vi "Add Dependency Dialog.vi"() -> (1 "Cancelled?":bool, 3 "Dependency Out":T3)   [LabVIEW 2015, in "Configuration Tool.lvlib"]
uses:
  XML Controls/Dependencies Properties.ctl
  XML Controls/Path Cluster.ctl
  XML Controls/Supported Targets.ctl
  Configuration Tool.lvlib
  VeriStand Custom Device XML Parser.lvlib
panel:
  in  "Cancel_Button":bool
  in  "OK_Button":bool
  in  "Path Properties":T1
  in  "Supported Target":T2
  in  "Supported Target Specified?":bool
  in  "Version":string
  in  "RealTimeSystemDestination":string
  in  "Force Download":bool
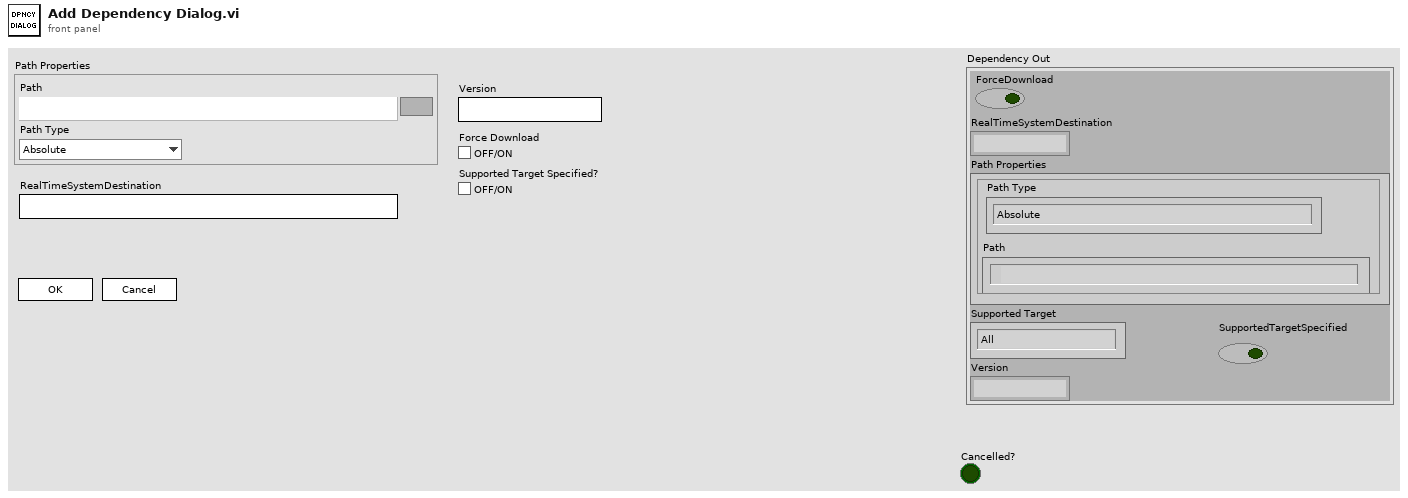
[diagram p1: front panel]
types:
  T1 = typedef "VeriStand Custom Device XML Parser.lvlib/Path Cluster.ctl" = cluster{"Path":path, "Path Type":enum16{"Absolute", "To Base", "To Common Doc Dir", "To Application Data Dir"}}
  T2 = typedef "VeriStand Custom Device XML Parser.lvlib/Supported Targets.ctl" = enum16{"All", "Pharlap", "VxWorks", "Windows", "Linux_32_ARM", "Linux_x64", "PharlapWindows", "PharlapVxWorks", "VxWorksWindows"}
  T3 = typedef "VeriStand Custom Device XML Parser.lvlib/Dependencies Properties.ctl" = cluster{"ForceDownload":bool, "RealTimeSystemDestination":string, "Path Properties":T1, "Supported Target":T2, "Version":string, "SupportedTargetSpecified":bool}
  T4 = enum32{"Invalid", "Standard", "Closed", "Hidden", "Minimized", "Maximized"}
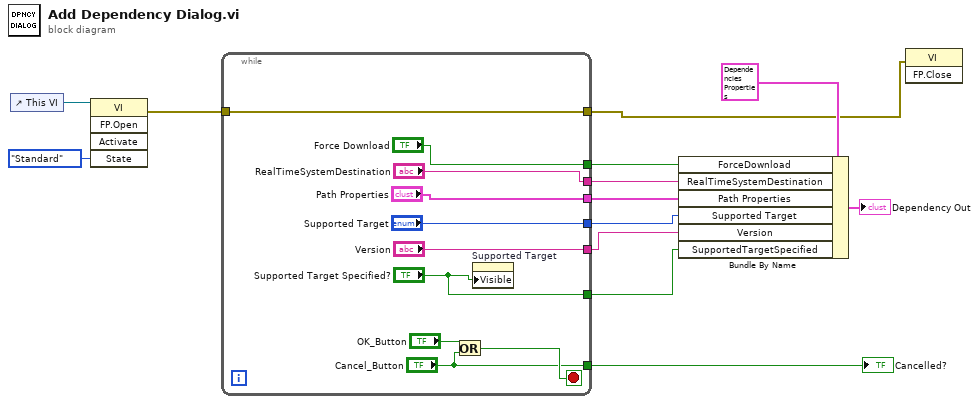
[diagram p0: block diagram]
diagram:
  n1 = control-ref of="This VI"() -> (w4:refnum<vi>)
  n2 = invoke class="VI" method="FP.Open"(reference=w4, "State"=T4."Standard") -> (error out=w3:errorcluster)  [unwired: 3 in, 4 out]
  n3 = while {
    tunnel: ["Force Download"] -> w11
    tunnel: ["RealTimeSystemDestination"] -> w10
    tunnel: ["Path Properties"] -> w9
    tunnel: ["Supported Target"] -> w8
    tunnel: ["Version"] -> w7
    tunnel: ["Supported Target Specified?"] -> w6
    tunnel: ["Cancel_Button"] -> w5
    tunnel: w3 -> [w14]
    tunnel: [w14] -> w2
    stop <- w16 stop-if-true
    n4 = Or(x="OK_Button", y="Cancel_Button") -> (x .or. y?=w16:bool)
    n5 = property on="Supported Target" class="Enum (strict)"("Visible"="Supported Target Specified?") -> ()  [unwired: 2 in, 2 out]
  }
  "Cancelled?" <- w5
  n6 = Bundle By Name(cluster=T3 {"ForceDownload"=FALSE, "RealTimeSystemDestination"="", "Path Properties"={"Path"=path "", "Path Type"=enum."Absolute"}, "Supported Target"=enum."All", "Version"="", "SupportedTargetSpecified"=FALSE} ("output cluster"), "ForceDownload"=w11, "RealTimeSystemDestination"=w10, "Path Properties"=w9, "Supported Target"=w8, "Version"=w7, "SupportedTargetSpecified"=w6) -> (→"Dependency Out":T3)
  n7 = invoke class="VI" method="FP.Close"(error in=w2) -> ()  [unwired: 2 in, 3 out]
